vi "Save Defaults.vi"() -> ()   [LabVIEW 2011]
panel:
  in  "Save?":bool
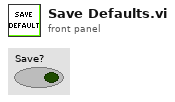
[diagram p1: front panel]
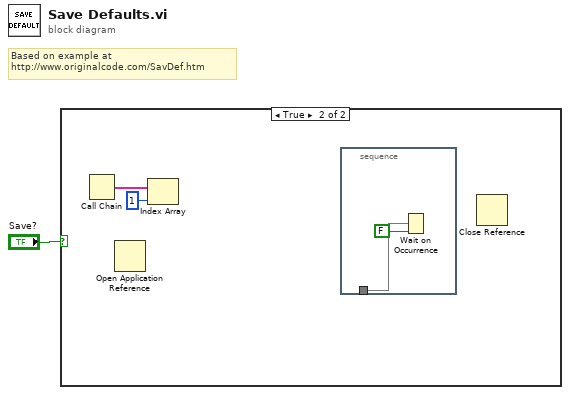
[diagram p0: block diagram]
diagram:
  # "Based on example at\nhttp://www.originalcode.com/SavDef.htm"
  n1 = case shown="True" "Save?" {
    frame False {
    }
    frame True {
      n2 = Call Chain() -> (call chain=w3:string[])
      n3 = Open Application Reference() -> ()  [unwired: 4 in, 2 out]
      n4 = Index Array(array=w3, index=1) -> ()  [unwired: 1 out]
      n5 = stacked-sequence {
        tunnel: _ -> [w4]
        frame #0 {
          n6 = Wait on Occurrence(1:FALSE ("ignore previous (T)"), 2:w4) -> ()  [unwired: 1 in, 1 out]
        }
      }
      n7 = Close Reference() -> ()  [unwired: 2 in, 1 out]
    }
  }
